vi "Get GMOD Library Path.vi"(8 "error in (no error)":errorcluster, 11 "VI in":refnum<vi>) -> (0 "error out":errorcluster, 3 "appended path":path)   [LabVIEW 2015, in "Generic Module Library.lvlib"]
uses:
  Generic Module Library.lvlib
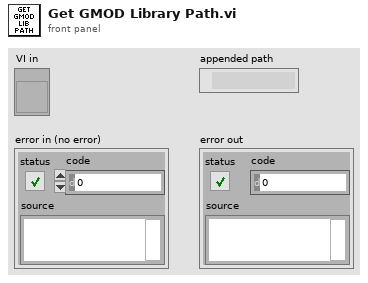
[diagram p1: front panel]
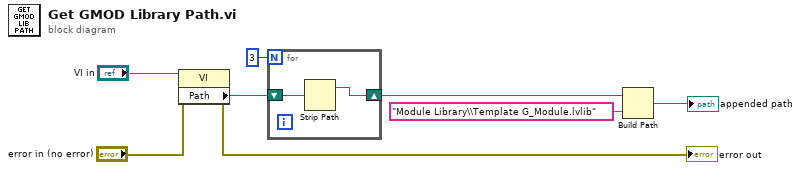
[diagram p0: block diagram]
diagram:
  n1 = property class="VI"(reference="VI in", error in="error in (no error)") -> (error out=→"error out":errorcluster, "Path"=w2:path)  [unwired: 1 out]
  n2 = for {
    N: 3 -> [_]
    shift-right: [w9] -> w5
    shift-left: w2 -> [w10]
    n3 = Strip Path(path=w10) -> (stripped path=w9:path)  [unwired: 1 out]
  }
  n4 = Build Path(base path=w5, name or relative path="Module Library\\Template G_Module.lvlib") -> (appended path=→"appended path":path)
